vi "Test MQTT-6.0.0-2.vi"(8 "error in (no error)":errorcluster, 11 "Connection Config":refnum<class "Connection.lvclass">) -> (0 "error out":errorcluster, 3 "Connection Config dup":refnum<class "Connection.lvclass">)   [LabVIEW 2013]
uses:
  <vilib>/addons/_JKI Toolkits/Caraya/classes/Test/Test.lvclass
  <vilib>/LabVIEW Open Source Project/Connection/Connection/Connection.lvclass
  <vilib>/LabVIEW Open Source Project/MQTT Websockets Connection/MQTT_Websockets/Connection/WebsocketsConnection.lvclass
  <vilib>/LabVIEW Open Source Project/MQTT Control Packets/Control Packets/CONNECT/CONNECT.lvclass
  <vilib>/LabVIEW Open Source Project/MQTT Control Packets/Control Packets/ControlPacket/ControlPacket.lvclass
  <vilib>/LabVIEW Open Source Project/MQTT Control Packets/Control Packets/ControlPacket/Control Packet Type -- enum.ctl
  <vilib>/LabVIEW Open Source Project/MQTT Control Packets/Control Packets/DISCONNECT/DISCONNECT.lvclass
  <vilib>/addons/_JKI Toolkits/Caraya/classes/Assert/Assert.lvclass
  <vilib>/LabVIEW Open Source Project/MQTT Connection/MQTT_Connection/Connection/Connection.lvclass
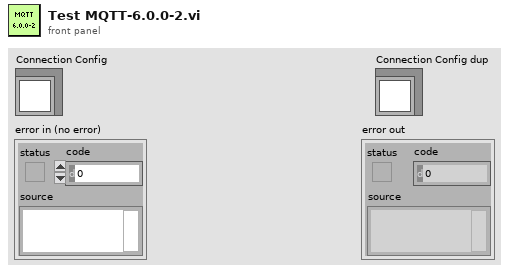
[diagram p1: front panel]
types:
  T1 = typedef "MQTT_Control_Packets.lvlib/ControlPacket.lvclass/Control Packet Type -- enum.ctl" = enum16{"Reserved", "CONNECT", "CONNACK", "PUBLISH", "PUBACK", "PUBREC", "PUBREL", "PUBCOMP", "SUBSCRIBE", "SUBACK", "UNSUBSCRIBE", "UNSUBACK", "PINGREQ", "PINGRESP", "DISCONNECT", "AUTH"}
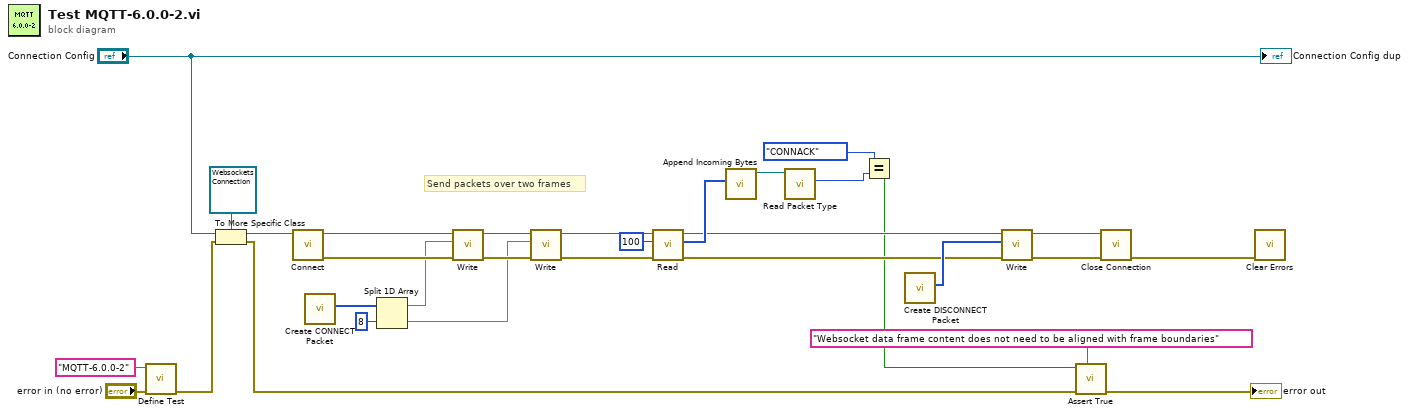
[diagram p0: block diagram]
diagram:
  # "Send packets over two frames"
  n1 = call <vilib>:"Define Test.vi"("error in (no error)"="error in (no error)", "Label (VI Title)"="MQTT-6.0.0-2") -> ("error out"=w23:errorcluster)  [unwired: 9 in]
  n2 = To More Specific Class(target class=refnum<class "WebsocketsConnection.lvclass"> refnum ("WebsocketsConnection in"), reference="Connection Config", error in=w23) -> (specific class reference=w25:refnum<class "WebsocketsConnection.lvclass">, error out=w22:errorcluster)
  n3 = call <vilib>:"Connect.vi"("Connection in"=w25) -> ("error out"=w20:errorcluster, "Connection out"=w21:refnum<class "WebsocketsConnection.lvclass">)  [unwired: 9 in]
  n4 = call <vilib>:"Create CONNECT Packet.vi"() -> ("Bytes Stream"=w11:u8[])  [unwired: 9 in, 2 out]
  n5 = Split 1D Array(array=w11, index=8) -> (first subarray=w12:u8[], second subarray=w13:u8[])
  n6 = call <vilib>:"Write.vi"("error in (no error)"=w20, "Bytes"=w12, "Connection in"=w21) -> ("error out"=w16:errorcluster, "Connection"=w18:refnum<class "WebsocketsConnection.lvclass">)  [unwired: 7 in]
  n7 = call <vilib>:"Write.vi"("error in (no error)"=w16, "Bytes"=w13, "Connection in"=w18) -> ("error out"=w15:errorcluster, "Connection"=w17:refnum<class "WebsocketsConnection.lvclass">)  [unwired: 7 in]
  n8 = call <vilib>:"Read.vi"("error in (no error)"=w15, "bytes to read (100)"=100, "TCPConnection in"=w17) -> ("error out"=w3:errorcluster, "Bytes"=w10:u8[], "TCPConnection out"=w5:refnum<class "WebsocketsConnection.lvclass">)  [unwired: 4 in, 2 out]
  n9 = call <vilib>:"Append Incoming Bytes.vi"("Incoming Packets"=w10) -> ("ControlPacket"=w9:refnum<class "ControlPacket.lvclass">)  [unwired: 7 in, 3 out]
  n10 = call <vilib>:"Read Packet Type.vi"("ControlPacket in"=w9) -> ("Control Packet Type"=w8:T1)  [unwired: 9 in, 1 out]
  n11 = Equal?(x=Control_Packet_Type_--_enum."CONNACK", y=w8) -> (x = y?=w1:bool)
  n12 = call <vilib>:"Create DISCONNECT Packet.vi"() -> ("Bytes Stream"=w6:u8[])  [unwired: 9 in, 2 out]
  n13 = call <vilib>:"Write.vi"("error in (no error)"=w3, "Bytes"=w6, "Connection in"=w5) -> ("error out"=w2:errorcluster, "Connection"=w4:refnum<class "WebsocketsConnection.lvclass">)  [unwired: 7 in]
  n14 = call <vilib>:"Assert True.vi"("Label"="Websocket data frame content does not need to be aligned with frame boundaries", "error in (no error)"=w22, "True?"=w1) -> ("error out"=→"error out":errorcluster)  [unwired: 8 in]
  n15 = call <vilib>:"Close Connection.vi"("error in (no error)"=w2, "Connection in"=w4) -> ("error out"=w26:errorcluster)  [unwired: 8 in, 1 out]
  n16 = call <vilib>:"Clear Errors.vi"("error in (no error)"=w26) -> ()  [unwired: 6 in, 1 out]
  "Connection Config dup" <- "Connection Config"
